vi "Lakeshore 336 Gen Channel names.vi"(11 "Lakeshore 336 Settings":T1={"Lake Shore 336 Address"="TCPIP0::192.168.121.12::7777::SOCKET", "Output Ch"=[], "Input Ch"=[], "Prefix"="", "Setpoints"=[], "Control Enable"=[]} {"Output Ch"."Heater Resistance (1:25 Ohms)" items=["25 Ohms"=1, "50 Ohms"=2]; "Output Ch"."Max User Current (2.000)" format="%.3f"; "Output Ch"."Heater Out Display (1:Current)" items=["Current"=1, "Power"=2]; "Output Ch"."Max Current (0:User Specified)" items=["User Specified", "0.707 A", "1.0 A", "1.141 A", "2.0 A"]; "Output Ch"."Mode (0:Off)" items=["Off", "Closed Loop PID", "Zone", "Open Loop"]; "Output Ch"."Input (0:None)" items=["None", "A", "B", "C", "D"]}) -> (2 "Channel Names":string[](array[string])=["Telescope RA", "Telescope DEC", "Telescope Moving?", "Telescope Status"], 3 "Channel List":refnum<class "HK Item.lvclass">[](array[class]))   [LabVIEW 2022 SP3, in "Lakeshore 336.lvclass"]
uses:
  Lakeshore 336.lvclass
  hk-channel-class/hk-channel-class/HK Item/HK Item.lvclass
  Lakeshore 336 Settings cluster.ctl
  Lakeshore 336 Channel Settings cluster.ctl
  Lakeshore 336 PID cluster.ctl
  Lakeshore 336 Input Ch config cluster.ctl
  hk-channel-class/hk-channel-class/HK Item/HK Channel Units and Setup.ctl
  hk-channel-class/hk-channel-class/HK Item/HK Channel enum Data Type.ctl
  Lakeshore 336.lvclass/Lakeshore 336.ctl
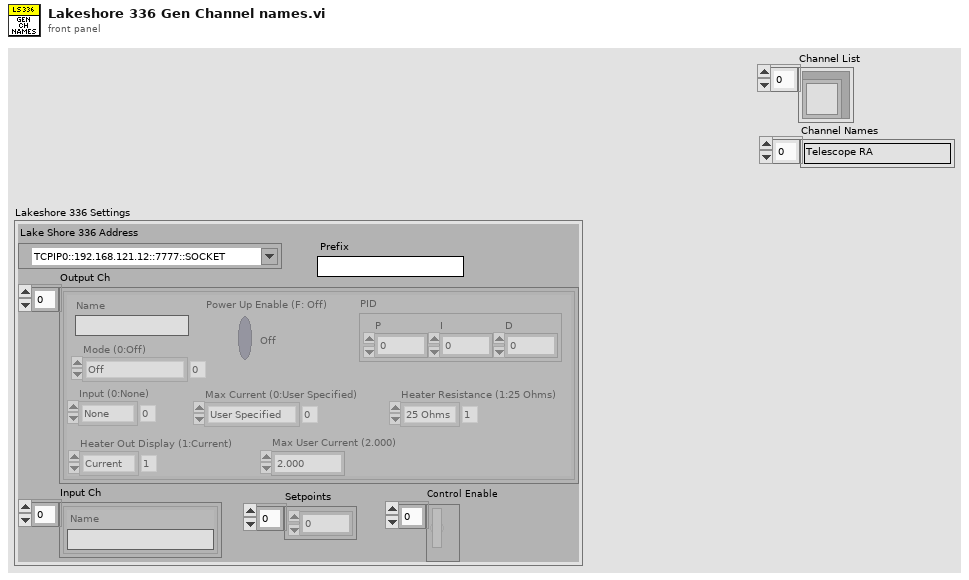
[diagram p1: front panel]
types:
  T1 = typedef "Lakeshore 336.lvclass/Lakeshore 336 Settings cluster.ctl" = cluster{"Lake Shore 336 Address":refnum<visa-resource-name>, "Output Ch":T2[], "Input Ch":T4[], "Prefix":string, "Setpoints":dbl[], "Control Enable":bool[]}
  T2 = typedef "Lakeshore 336.lvclass/Lakeshore 336 Channel Settings cluster.ctl" = cluster{"Input (0:None)":u16, "Power Up Enable (F: Off)":bool, "Mode (0:Off)":u16, "Max Current (0:User Specified)":u16, "Heater Out Display (1:Current)":u16, "Max User Current (2.000)":dbl, "Heater Resistance (1:25 Ohms)":u16, "PID":T3, "Name":string}
  T3 = typedef "Lakeshore 336.lvclass/Lakeshore 336 PID cluster.ctl" = cluster{"P":dbl, "I":dbl, "D":dbl}
  T4 = typedef "Lakeshore 336.lvclass/Lakeshore 336 Input Ch config cluster.ctl" = cluster{"Name":string}
  T5 = typedef "HK Item.lvclass/HK Channel Units and Setup.ctl" = cluster{"Unit Type":string, "Units":string, "Configuration":string, "Digits":i32, "Data Type":T6, "Exponential?":bool, "Source":string}
  T6 = typedef "HK Item.lvclass/HK Channel enum Data Type.ctl" = enum16{"Floating Point", "Integer", "Enum", "String", "Waveform", "File"}
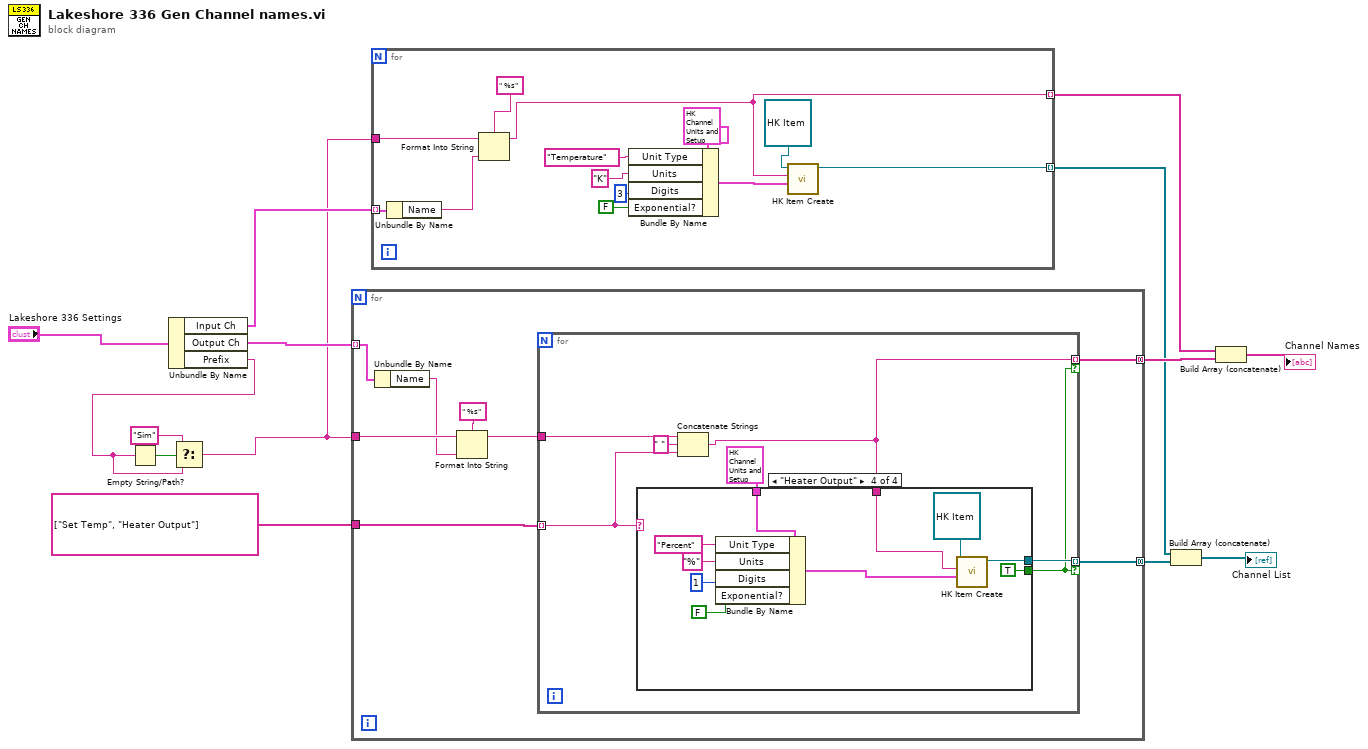
[diagram p0: block diagram]
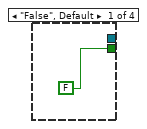
[diagram p2: hidden frame]
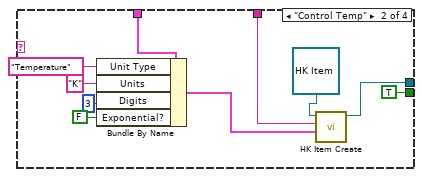
[diagram p3: hidden frame]
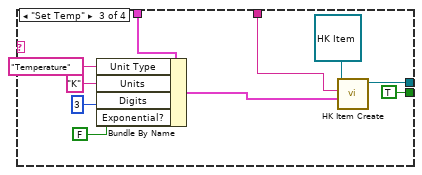
[diagram p4: hidden frame]
diagram:
  n1 = Unbundle By Name("Lakeshore 336 Settings") -> ("Input Ch"=w7:T4[], "Output Ch"=w8:T2[], "Prefix"=w1:string)
  n2 = Empty String/Path?(string/path=w1) -> (empty?=w11:bool)
  n3 = Select(t="Sim", s=w11, f=w1) -> (s? t:f=w6:string)
  n4 = for {
    tunnel: string[] ["Set Temp", "Heater Output"] -> [w22]
    tunnel: [w21] -> w13 mode=concatenating
    tunnel: [w20] -> w12 mode=concatenating
    tunnel: w6 -> [w17]
    tunnel: w8 -> [w19] mode=indexing
    n5 = Unbundle By Name(w19) -> ("Name"=w16:string)
    n6 = Format Into String(format string=" %s", initial string=w17, w16) -> (resulting string=w15:string)  [unwired: 1 in, 1 out]
    n7 = for {
      tunnel: w22 -> [w27] mode=indexing
      tunnel: [w25] -> w20 mode=indexing if=w24
      tunnel: [w23] -> w21 mode=indexing if=w24
      tunnel: w15 -> [w28]
      n8 = Concatenate Strings(w28, " " ("string"), w27) -> (w23:string)
      n9 = case shown="\"Heater Output\"" w27 {
        tunnel: T5 {"Unit Type"="", "Units"="", "Configuration"="", "Digits"=3, "Data Type"=enum."Floating Point", "Exponential?"=FALSE, "Source"=""} ("Channel Setup") -> [_ w40 w50 w60]
        tunnel: w23 -> [_ w33 w44 w54]
        tunnel: [_ w32 w42 w52] -> w25
        tunnel: [FALSE TRUE TRUE TRUE] -> w24
        frame "False", Default {
        }
        frame "Control Temp" {
          n10 = Bundle By Name(cluster=w40, "Unit Type"="Temperature", "Units"="K", "Digits"=3, "Exponential?"=FALSE) -> (w34:T5)
          n11 = call-dynamic "HK Item Create.vi"("Channel Setup"=w34, "Name"=w33, "HK Item in"=refnum<class "HK Item.lvclass"> refnum) -> ("HK Item out"=w32:refnum<class "HK Item.lvclass">)  [unwired: 7 in, 1 out]
        }
        frame "Set Temp" {
          n12 = Bundle By Name(cluster=w50, "Unit Type"="Temperature", "Units"="K", "Digits"=3, "Exponential?"=FALSE) -> (w45:T5)
          n13 = call-dynamic "HK Item Create.vi"("Channel Setup"=w45, "Name"=w44, "HK Item in"=refnum<class "HK Item.lvclass"> refnum) -> ("HK Item out"=w42:refnum<class "HK Item.lvclass">)  [unwired: 7 in, 1 out]
        }
        frame "Heater Output" {
          n14 = Bundle By Name(cluster=w60, "Unit Type"="Percent", "Units"="%", "Digits"=1, "Exponential?"=FALSE) -> (w55:T5)
          n15 = call-dynamic "HK Item Create.vi"("Channel Setup"=w55, "Name"=w54, "HK Item in"=refnum<class "HK Item.lvclass"> refnum) -> ("HK Item out"=w52:refnum<class "HK Item.lvclass">)  [unwired: 7 in, 1 out]
        }
      }
    }
  }
  n16 = for {
    tunnel: w7 -> [w68] mode=indexing
    tunnel: w6 -> [w67]
    tunnel: [w62] -> w4 mode=indexing
    tunnel: [w61] -> w2 mode=indexing
    n17 = Unbundle By Name(w68) -> ("Name"=w66:string)
    n18 = Format Into String(format string=" %s", initial string=w67, w66) -> (resulting string=w61:string)  [unwired: 1 in, 1 out]
    n19 = Bundle By Name(cluster=T5 {"Unit Type"="", "Units"="", "Configuration"="", "Digits"=3, "Data Type"=enum."Floating Point", "Exponential?"=FALSE, "Source"=""} ("Channel Setup"), "Unit Type"="Temperature", "Units"="K", "Digits"=3, "Exponential?"=FALSE) -> (w71:T5)
    n20 = call-dynamic "HK Item Create.vi"("Channel Setup"=w71, "Name"=w61, "HK Item in"=refnum<class "HK Item.lvclass"> refnum) -> ("HK Item out"=w62:refnum<class "HK Item.lvclass">)  [unwired: 7 in, 1 out]
  }
  n21 = Build Array (concatenate)(w4, w12) -> (→"Channel List":refnum<class "HK Item.lvclass">[])
  n22 = Build Array (concatenate)(w2, w13) -> (→"Channel Names":string[])
